vi "Import VI Snippet read PNG.vi"(8 "error in (no error)":errorcluster, 11 "Path (*.png)":path) -> (0 "error out":errorcluster, 3 "Chunks":T1(array[cluster]) {"CRC" format="%08x"})   [LabVIEW 2019]
doc: "Returns the PNG image chunks from the <b>Path</b>.\n\nCreated by: Ryan Pacini"
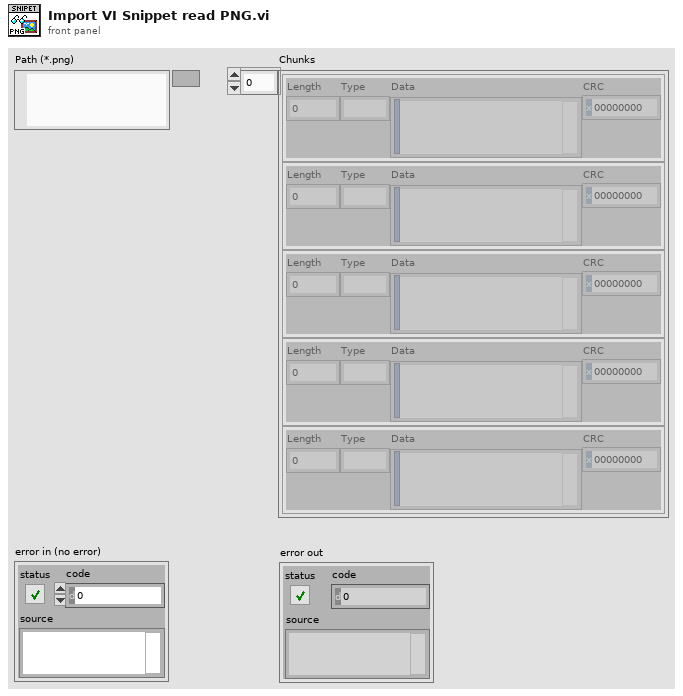
[diagram p1: front panel]
types:
  T1 = cluster{"Length":i32, "Type":string, "Data":string, "CRC":u32}[]
  T2 = cluster{"Length":i32, "Type":string, "Data":string, "CRC":u32}
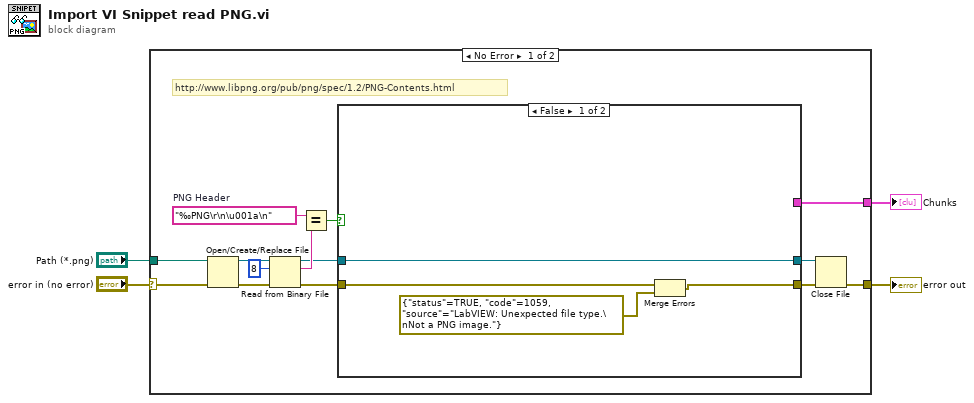
[diagram p0: block diagram]
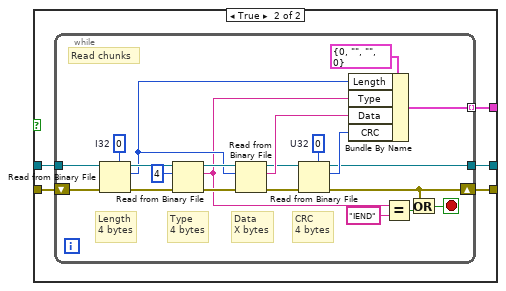
[diagram p2: hidden frame]
diagram:
  n1 = case shown="No Error" "error in (no error)" {
    selector: "error in (no error)" -> [w18 w50]
    tunnel: "Path (*.png)" -> [w17 _]
    tunnel: [w11 _] -> w2
    tunnel: [w9 w50] -> w1
    frame No Error {
      w5 = "‰PNG\r\n\u001a\n"  # PNG Header
      # "http://www.libpng.org/pub/png/spec/1.2/PNG-Contents.html"
      n2 = Open/Create/Replace File(file path (use dialog)=w17, error in=w18) -> (refnum out=w16:refnum<file>, error out=w15:errorcluster)  [unwired: 4 in, 1 out]
      n3 = Read from Binary File(8:w15, 10:8 ("count (1)"), 11:w16) -> (0:w13:errorcluster, 2:w14:string, 3:w12:refnum<file>)  [unwired: 3 in, 1 out]
      n4 = Equal?(x=w5, y=w14) -> (x = y?=w7:bool)
      n5 = case shown="False" w7 {
        tunnel: w13 -> [w21 w27]
        tunnel: w12 -> [w22 w26]
        tunnel: [_ w25] -> w11
        tunnel: [w20 w24] -> w10
        tunnel: [w22 w23] -> w8
        frame False {
          n6 = Merge Errors(w21, errorcluster {"status"=TRUE, "code"=1059, "source"="LabVIEW: Unexpected file type.\nNot a PNG image."} ("error in")) -> (w20:errorcluster)
        }
        frame True {
          n7 = while {
            tunnel: w26 -> [w48]
            tunnel: [w45] -> w25 mode=indexing
            shift-right: [w33] -> w24
            shift-left: w27 -> [w49]
            tunnel: [w29] -> w23
            stop <- w30 stop-if-true
            w35 = u32 0  # U32
            w47 = 0  # I32
            # "Read chunks"
            # "CRC\n4 bytes"
            # "Data\nX bytes"
            # "Type\n4 bytes"
            # "Length\n4 bytes"
            n8 = Read from Binary File(5:w47, 8:w49, 11:w48) -> (0:w44:errorcluster, 2:w39:i32, 3:w43:refnum<file>)  [unwired: 3 in, 1 out]
            n9 = Read from Binary File(8:w44, 10:4 ("count (1)"), 11:w43) -> (0:w41:errorcluster, 2:w32:string, 3:w40:refnum<file>)  [unwired: 3 in, 1 out]
            n10 = Read from Binary File(8:w41, 10:w39, 11:w40) -> (0:w37:errorcluster, 2:w38:string, 3:w36:refnum<file>)  [unwired: 3 in, 1 out]
            n11 = Read from Binary File(5:w35, 8:w37, 11:w36) -> (0:w33:errorcluster, 2:w34:u32, 3:w29:refnum<file>)  [unwired: 3 in, 1 out]
            n12 = Bundle By Name(cluster=T2 {"Length"=0, "Type"="", "Data"="", "CRC"=0} ("Chunks"), "Length"=w39, "Type"=w32, "Data"=w38, "CRC"=w34) -> (w45:T2)
            n13 = Equal?(x=w32, y="IEND") -> (x = y?=w31:bool)
            n14 = Or(x=w33, y=w31) -> (x .or. y?=w30:bool)
          }
        }
      }
      n15 = Close File(refnum=w8, error in=w10) -> (error out=w9:errorcluster)  [unwired: 1 out]
    }
    frame Error {
    }
  }
  "error out" <- w1
  "Chunks" <- w2
